vi "GetDiagramSubVIs.vi"(5 "Diagram":refnum<class "Diagram.lvclass">, 6 "error in":errorcluster, 9 "VI Interpreter in":refnum<class "VI Interpreter.lvclass">) -> (0 "error out":errorcluster, 3 "VI Interpreter out":refnum<class "VI Interpreter.lvclass">, 4 "Diagram out":refnum<class "Diagram.lvclass">)   [LabVIEW 2014, in "Raspberry Pi Compatible Compiler for LabVIEW.lvlib" / "VI Interpreter.lvclass"]
uses:
  VI Interpreter.lvclass
  Diagram/Diagram.lvclass
  Diagram/Diagram.lvclass/Diagram.ctl
  SubVI/SubVI.lvclass
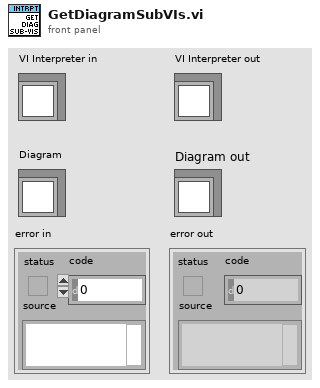
[diagram p1: front panel]
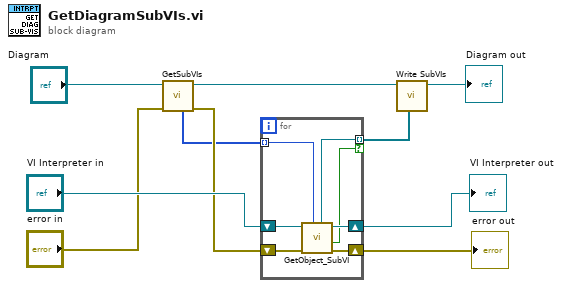
[diagram p0: block diagram]
diagram:
  n1 = call "GetSubVIs.vi"("error in"="error in", "Diagram in"="Diagram") -> ("error out"=w5:errorcluster, "Diagram out"=w3:refnum<class "Diagram.lvclass">, "subVIs"=w4:i32[])  [unwired: 5 in]
  n2 = for {
    shift-right: [w14] -> w10
    shift-left: "VI Interpreter in" -> [w17]
    shift-right: [w16] -> w9
    shift-left: w5 -> [w15]
    tunnel: [w13] -> w2 mode=indexing if=w12
    tunnel: w4 -> [w11] mode=indexing
    n3 = call "GetObject_SubVI.vi"("UID"=w11, "error in"=w15, "VI Interpreter in"=w17) -> ("error out"=w16:errorcluster, "found"=w12:bool, "VI Interpreter out"=w14:refnum<class "VI Interpreter.lvclass">, "SubVI out"=w13:refnum<class "SubVI.lvclass">)  [unwired: 3 in]
  }
  "error out" <- w9
  "VI Interpreter out" <- w10
  n4 = call "Write SubVIs.vi"("SubVIs"=w2, "Diagram in"=w3) -> ("Diagram out"=→"Diagram out":refnum<class "Diagram.lvclass">)  [unwired: 7 in]
